vi "gradient_fi.vi"(1 "q_input":dbl[](array[numeric]), 2 "constraints cluster":T1) -> (0 "gradient of fi":dbl[][](array[numeric]))   [LabVIEW 2019]
panel:
  # "input : constraints cluster\n             q_input"
  # "output : gradient of fi, \n               matrix\n               n*m"
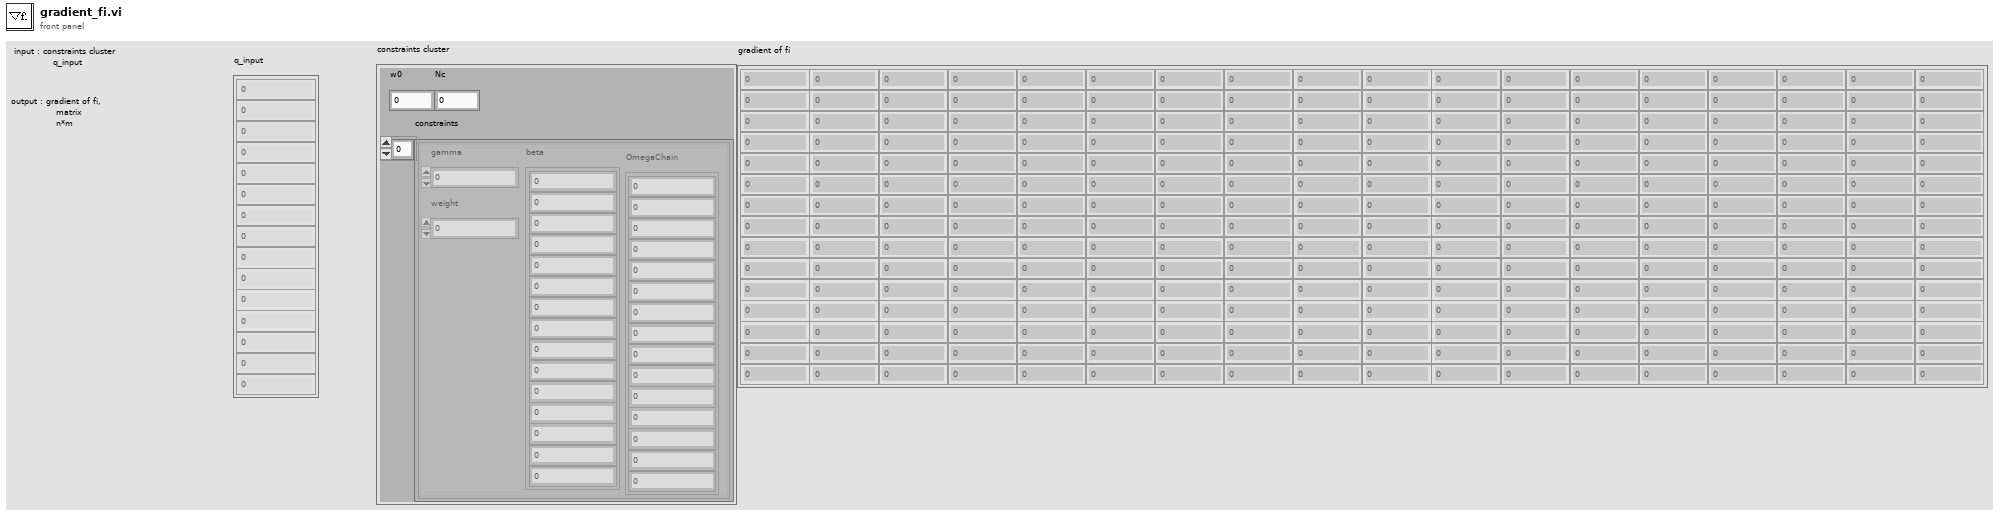
[diagram p1: front panel]
types:
  T1 = cluster{"w0":dbl, "constraints":cluster{"beta":dbl[], "gamma":dbl, "OmegaChain":dbl[], "weight":dbl}[], "Nc":i32}
  T2 = cluster{"beta":dbl[], "gamma":dbl, "OmegaChain":dbl[], "weight":dbl}[]
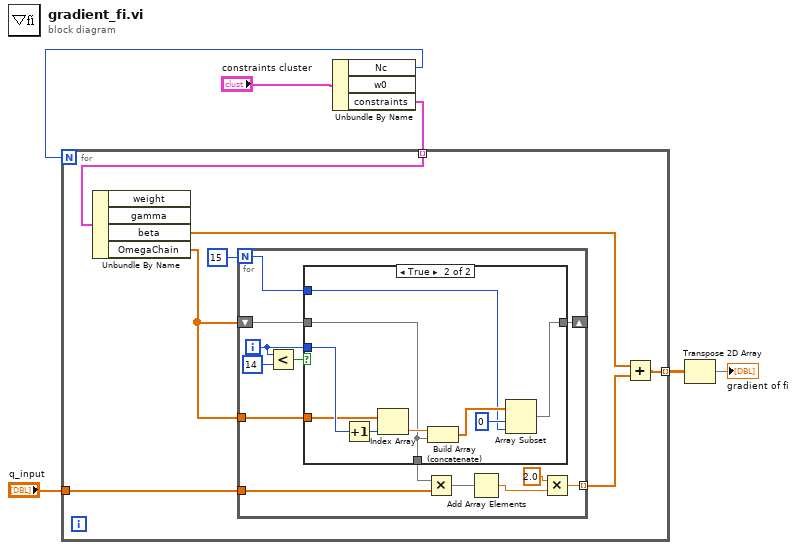
[diagram p0: block diagram]
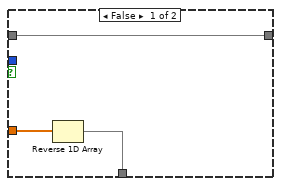
[diagram p2: hidden frame]
diagram:
  n1 = Unbundle By Name("constraints cluster") -> ("Nc"=w4:i32, "constraints"=w3:T2)  [unwired: 1 out]
  n2 = for {
    N: w4 -> [_]
    tunnel: "q_input" -> [w9]
    tunnel: [w7] -> w2 mode=indexing
    tunnel: w3 -> [w12] mode=indexing
    n3 = Unbundle By Name(w12) -> ("beta"=w13:dbl[], "OmegaChain"=w10:dbl[])  [unwired: 2 out]
    n4 = for {
      N: 15 -> [w23]
      tunnel: w9 -> [w26]
      tunnel: [w15] -> w8 mode=indexing
      tunnel: w10 -> [w19]
      shift-right: [w16] -> _
      shift-left: w10 -> [w17]
      i -> [w20]
      n5 = Less?(x=w20, y=14) -> (x < y?=w21:bool)
      n6 = case shown="True" w21 {
        tunnel: w20 -> [_ w34]
        tunnel: w23 -> [_ w33]
        tunnel: w19 -> [w29 w32]
        tunnel: [w28 w31] -> w18
        tunnel: w17 -> [w27 w31]
        tunnel: [w27 w30] -> w16
        frame False {
          n7 = Reverse 1D Array(array=w29) -> (reversed array=w28:dbl[])
        }
        frame True {
          n8 = Increment(x=w34) -> (x+1=w35:i32)
          n9 = Index Array(array=w32, index=w35) -> (element=w36:dbl)
          n10 = Build Array (concatenate)(w36, w31) -> (w37:dbl[])
          n11 = Array Subset(array=w37, index=0, length=w33) -> (w30:dbl[])
        }
      }
      n12 = Multiply(x=w18, y=w26) -> (x*y=w25:dbl[])
      n13 = Add Array Elements(numeric array=w25) -> (sum=w24:dbl)
      n14 = Multiply(x=2.0, y=w24) -> (x*y=w15:dbl)
    }
    n15 = Add(x=w13, y=w8) -> (x+y=w7:dbl[])
  }
  n16 = Transpose 2D Array(2D array=w2) -> (transposed array=→"gradient of fi":dbl[][])
